vi "DevB.Close Message Session.vi"(8 "error in":errorcluster, 11 "DevBoard Message session":T1) -> (0 "error out":errorcluster)   [LabVIEW 2018]
uses:
  typedefs/DevB.Message Session.ctl
  typedefs/DevB.Message.ctl
  typedefs/DevB.Message type.ctl
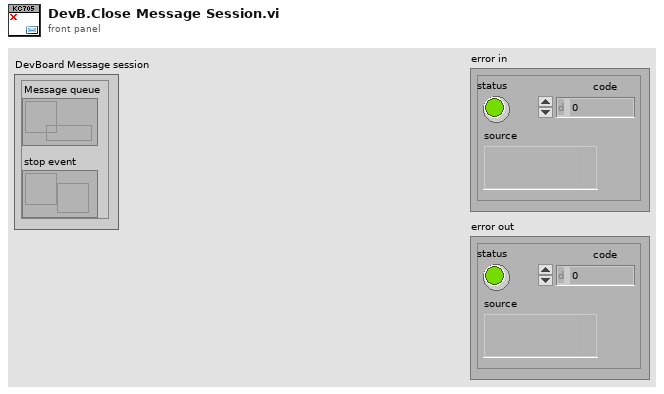
[diagram p1: front panel]
types:
  T1 = typedef "DevB.Message Session.ctl" = cluster{"Message queue":refnum<queue>, "stop event":refnum<user-event>}
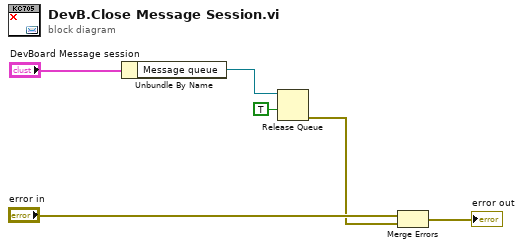
[diagram p0: block diagram]
diagram:
  n1 = Unbundle By Name("DevBoard Message session") -> ("Message queue"=w3:refnum<queue>)
  n2 = Release Queue(queue=w3, force destroy? (F)=TRUE) -> (error out=w2:errorcluster)  [unwired: 1 in, 2 out]
  n3 = Merge Errors("error in", w2) -> (→"error out":errorcluster)
